vi "Adjust Shooter.vi"(5 "Distance from end of cannon to center of target [Meter]":dbl, 6 "Upside Down?":bool, 7 "Start to Adjust":bool) -> (0 "Second Cannon":dbl, 1 "First Cannon":dbl, 2 "Cannon Angle":dbl, 3 "READY!":bool)   [LabVIEW 2012]
uses:
  BotStatus.vi
  <vilib>/express/express arith-compare/Formula/XNode/ExpressFormulaBlockNode.xnode
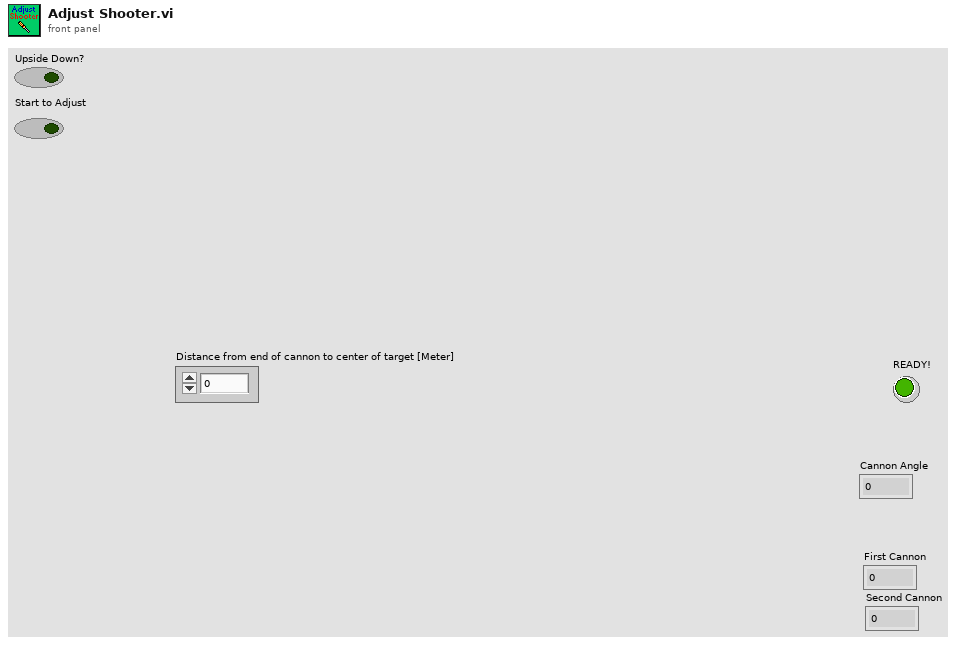
[diagram p1: front panel]
types:
  T1 = typedef "WPI_EncoderDevRef.ctl" = cluster{"DevStatus":errorcluster, "EncoderIndex":T2, "CounterIndex":T3, "DistancePerCount":dbl, "Decoding Type":T4}
  T2 = typedef "FPGA_EncoderIdx.ctl" = enum8{"Enc 0", "Enc 1", "Enc 2", "Enc 3", "Invalid"}
  T3 = typedef "FPGA_CounterCtrSystemIndex.ctl" = enum8{"Ctr 0", "Ctr 1", "Ctr 2", "Ctr 3", "Ctr 4", "Ctr 5", "Ctr 6", "Ctr 7", "Invalid"}
  T4 = typedef "WPI_EncoderType.ctl" = enum16{"1x", "2x", "4x"}
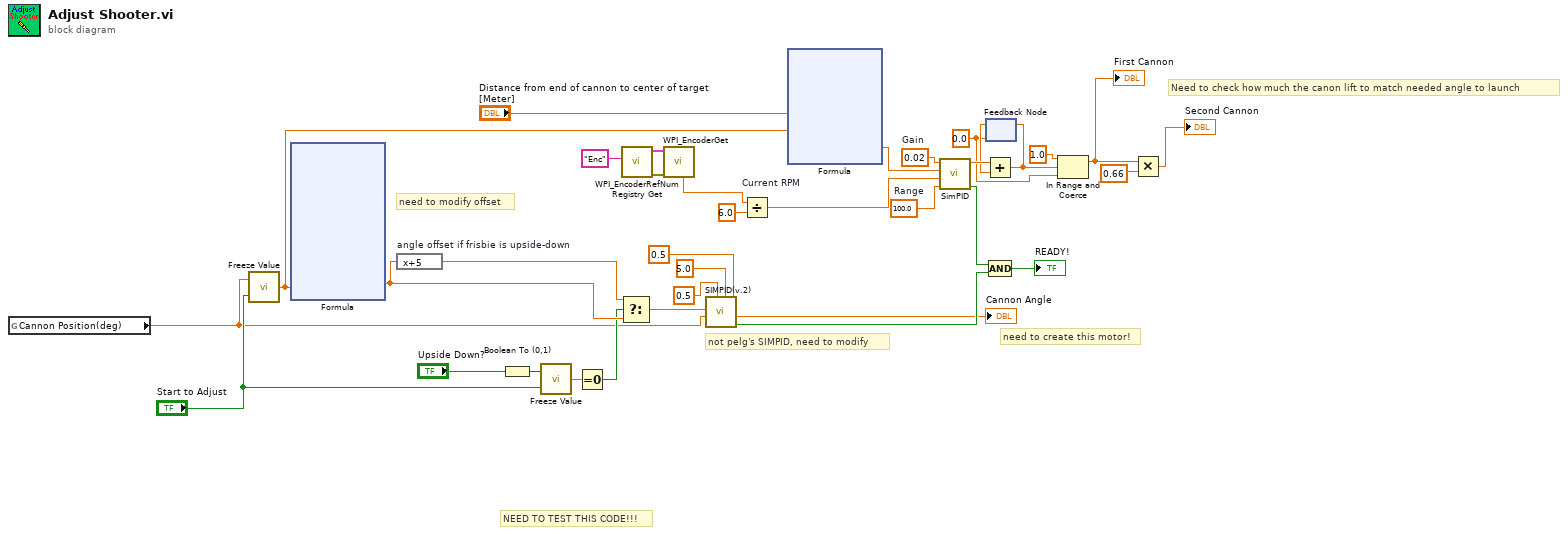
[diagram p0: block diagram]
diagram:
  w11 = 0.0
  w20 = 100.0  # Range
  w21 = 0.02  # Gain
  # "NEED TO TEST THIS CODE!!!"
  # "Need to check how much the canon lift to match needed angle to launch"
  # "need to create this motor!"
  # "need to modify offset"
  # "not pelg's SIMPID, need to modify"
  n1 = global read "BotStatus.vi" "Cannon Position(deg)"() -> (w1:dbl)
  n2 = call "Freeze Value.vi"("Freeze Value"="Start to Adjust", "In Value"=w1) -> ("Value Out"=w7:dbl)
  n3 = xnode "Formula"("angle"=w7) -> ("Result"=w9:dbl)  [unwired: 4 in, 1 out]
  n4 = expression code="x+5" "angle offset if frisbie is upside-down"(w9) -> (w8:dbl)
  n5 = Boolean To (0,1)(Boolean="Upside Down?") -> (0, 1=w4:i16)
  n6 = call "Freeze Value.vi"("Freeze Value"="Start to Adjust", "In Value"=w4) -> ("Value Out"=w3:dbl)
  n7 = Equal To 0?(x=w3) -> (x = 0?=w2:bool)
  n8 = Select(t=w8, s=w2, f=w9) -> (s? t:f=w10:dbl)
  n9 = call <vilib>:"WPI_EncoderRefNum Registry Get.vi"("refnum name"="Enc") -> ("error out"=w26:errorcluster, "EncoderDevRef"=w27:T1)  [unwired: 9 in]
  n10 = call <vilib>:"WPI_EncoderGet.vi"("error in (no error)"=w26, "EncoderDevRef"=w27) -> ("Rate"=w24:dbl)  [unwired: 4 in, 5 out]
  n11 = call "SIMPID(v.2).vi"("Range"=0.5, "upper limit"=5.0, "lower limit"=0.5, "Current Point"=w1, "Set Point"=w10) -> ("On Target"=w32:bool, "result"=→"Cannon Angle":dbl)  [unwired: 5 in]
  n12 = Divide "Current RPM"(x=w24, y=6.0) -> (x/y=w19:dbl)
  n13 = xnode "Formula"("D"="Distance from end of cannon to center of target [Meter]", "angle"=w7) -> ("Result"=w18:dbl)  [unwired: 1 in, 1 out]
  n14 = call "SimPID.vi"("Range"=w20, "Position"=w19, "Set Point"=w18, "Gain"=w21) -> ("On Target"=w17:bool, "result"=w16:dbl)  [unwired: 5 in]
  n15 = feedback #1(w11) -> (w15:dbl)
  n16 = Add(x=w16, y=w15) -> (x+y=w14:dbl)
  n17 = feedback-in #1(w14) -> ()
  n18 = Compound Arithmetic op=AND(w17, w32) -> (→"READY!":bool)
  n19 = In Range and Coerce(upper limit=1.0, x=w14, lower limit=w11) -> (coerced(x)=w13:dbl)  [unwired: 1 out]
  "First Cannon" <- w13
  n20 = Multiply(x=w13, y=0.66) -> (x*y=→"Second Cannon":dbl)
